vi "VSI Flash Write Bytes.vi"(6 "WriteLen":u16, 7 "pWriteData":string, 8 "error in (no error)":errorcluster, 9 "PageAddr":i32, 10 "DevIndex":i32, 11 "DevType":i32) -> (0 "error out":errorcluster, 3 "function return":i32)   [LabVIEW 2012, in "ControlSPI.lvlib"]
doc: "int WINAPI VSI_FlashWriteBytes(int DevType,int DevIndex,int PageAddr,unsigned char *pWriteData,unsigned short WriteLen);"
uses:
  ControlSPI.lvlib
  Ginkgo_Driver.dll
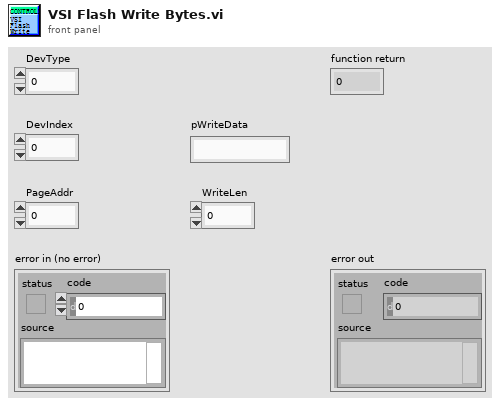
[diagram p1: front panel]
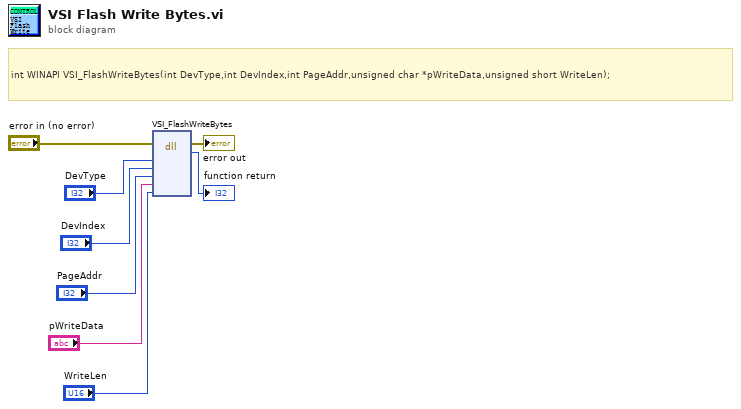
[diagram p0: block diagram]
diagram:
  # "int WINAPI VSI_FlashWriteBytes(int DevType,int DevIndex,int PageAddr,unsigned char *pWriteData,unsigned short WriteLen);"
  n1 = dll-call lib="E:/Project/vt_ginkgo/truck/Ginkgo Driver/vs2010/Ginkgo_USB-I2C_API_v2.0.3.0/lib/labview_32bit/ControlSPI/Ginkgo_Driver.*" fn="VSI_FlashWriteBytes"(error in="error in (no error)", "DevType"="DevType", "DevIndex"="DevIndex", "PageAddr"="PageAddr", "pWriteData"="pWriteData", "WriteLen"="WriteLen") -> (error out=→"error out":errorcluster, →"function return":i32)  [unwired: 7 in, 1 out]
